vi "Show Tree.vi"(7 "Root ID":string, 8 "Error In":errorcluster, 9 "Show IDs (False)":bool, 10 "Tree Ref":refnum<vi>, 11 "Tree":T1) -> (0 "Error Out":errorcluster, 3 "Tree":T1)   [LabVIEW 2020, in "NI_VIAnCFGDataStructure.lvlib" / "Tree.lvclass"]
doc: "Recursively traverse down wired Tree ID and populate the Tree Control with the contents of the Tree.\n\nBecause the Tree Control requires to have only one root element, the Root ID has to be specified. This means that if you have multiple roots in your Tree you need to visualize them seperately."
uses:
  <vilib>/addons/analyzer/VIAnCFGDataStructure/Tree Manager/Tree.lvclass
  <vilib>/addons/analyzer/VIAnCFGDataStructure/Tree Manager/Typedefs/Session Handle.ctl
  <vilib>/addons/analyzer/VIAnCFGDataStructure/Tree Manager/Tree.lvclass/Tree.ctl
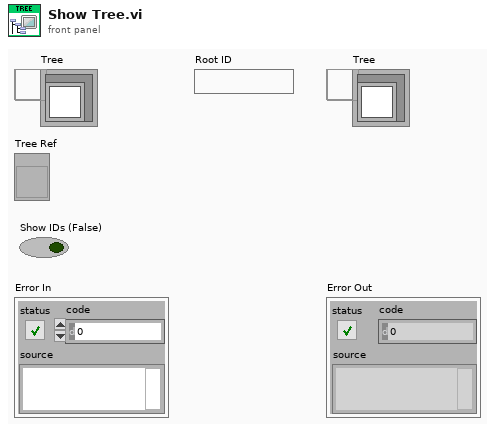
[diagram p1: front panel]
types:
  T1 = typedef "NI_VIAnCFGDataStructure.lvlib/Tree.lvclass/Session Handle.ctl" = refnum<data-value>
  T2 = cluster{"Left Cell String":string, "Child Text":string[], "Child Tag":string, "Item Indent":i32, "Child Only?":bool, "Glyph Index":i32}[]
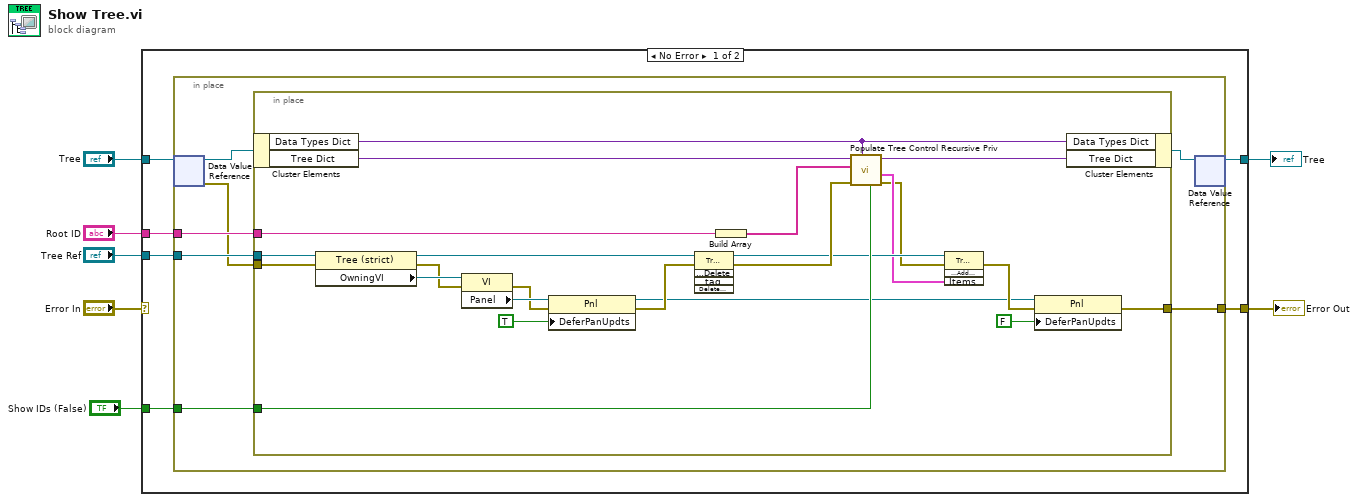
[diagram p0: block diagram]
diagram:
  n1 = case shown="No Error" "Error In" {
    selector: "Error In" -> [_ w44]
    tunnel: "Tree" -> [w13 w45]
    tunnel: [w12 w45] -> w6
    tunnel: [w9 w44] -> w4
    tunnel: "Root ID" -> [w11 _]
    tunnel: "Tree Ref" -> [w10 _]
    tunnel: "Show IDs (False)" -> [w8 _]
    frame No Error {
      n2 = in-place {
        in-place-border: w11 -> [w18]
        in-place-border: w10 -> [w16]
        in-place-border: [w17] -> w9
        in-place-border: w8 -> [w14]
        n3 = in-place-dvr #1(w13) -> (w20:refnum<class "Tree.lvclass">, w15:errorcluster)
        n4 = in-place {
          in-place-border: w18 -> [w40]
          in-place-border: [w29] -> w17
          in-place-border: w16 -> [w38]
          in-place-border: w15 -> [w37]
          in-place-border: w14 -> [w27]
          n5 = in-place-cluster #2(w20) -> ("Data Types Dict"=w26:variant, "Tree Dict"=w43:variant)
          n6 = property class="Tree (strict)"(reference=w38, error in=w37) -> (reference out=w32:refnum<vi>, error out=w35:errorcluster, "OwningVI"=w36:refnum<vi>)
          n7 = property class="VI"(reference=w36, error in=w35) -> (error out=w33:errorcluster, "Panel"=w34:refnum<vi>)  [unwired: 1 out]
          n8 = property class="Pnl"(reference=w34, error in=w33, "DeferPanUpdts"=TRUE ("Defer Panel Updates")) -> (reference out=w21:refnum<vi>, error out=w31:errorcluster)
          n9 = invoke class="Tree (strict)" method="Edit Tree Items.Delete"(reference=w32, error in=w31) -> (reference out=w25:refnum<vi>, error out=w41:errorcluster)  [unwired: 3 in, 3 out]
          n10 = Build Array(w40) -> (w39:string[])
          n11 = call <vilib>:"Populate Tree Control Recursive Priv.vi"("Show IDs (True)"=w27, "Data Types Dict"=w26, "error in"=w41, "Child IDs"=w39, "Tree Dictionary In"=w43) -> ("error out"=w23:errorcluster, "Items Out"=w24:T2, "Tree Dictionary Out"=w42:variant)  [unwired: 4 in]
          n12 = invoke class="Tree (strict)" method="Edit Tree Items.Add Multiple Items to End"(reference=w25, error in=w23, "Items"=w24) -> (error out=w22:errorcluster)  [unwired: 1 in, 3 out]
          n13 = property class="Pnl"(reference=w21, error in=w22, "DeferPanUpdts"=FALSE ("Defer Panel Updates")) -> (error out=w29:errorcluster)  [unwired: 1 out]
          n14 = in-place-cluster #2("Data Types Dict"=w26, "Tree Dict"=w42) -> (w19:refnum<class "Tree.lvclass">)
        }
        n15 = in-place-dvr #1(w19) -> (w12:T1)  [unwired: 1 out]
      }
    }
    frame Error {
    }
  }
  "Tree" <- w6
  "Error Out" <- w4
